vi "multi-function-fpga-main-Rev5.vi"(9 "stop":bool, 10 "Update":bool, 11 "fpga controls":T1[](array[typedef])=[{"Operation"=0, "Num. Steps"=0, "Begin"=0.0, "Step Size"=0.0, "Input - A"=0, "Input - B"=0, "Output - LO"=0.0, "Output - HI"=0.0, "Reset"=FALSE, "Analog Output"=0, "Trigger Input"=0, "Initialize To"=0, "Digital Inputs"=[0, 0, 0, 0, 0], "Output Values"=[0.0, 0.0, 0.0, 0.0, 0.0], "Num. Inputs"=4}, {"Operation"=0, "Num. Steps"=0, "Begin"=0.0, "Step Size"=0.0, "Input - A"=0, "Input - B"=0, "Output - LO"=0.0, "Output - HI"=0.0, "Reset"=FALSE, "Analog Output"=1, "Trigger Input"=0, "Initialize To"=0, "Digital Inputs"=[0, 0, 0, 0, 0], "Output Values"=[0.0, 0.0, 0.0, 0.0, 0.0], "Num. Inputs"=4}, {"Operation"=0, "Num. Steps"=0, "Begin"=0.0, "Step Size"=0.0, "Input - A"=0, "Input - B"=0, "Output - LO"=0.0, "Output - HI"=0.0, "Reset"=FALSE, "Analog Output"=2, "Trigger Input"=0, "Initialize To"=0, "Digital Inputs"=[0, 0, 0, 0, 0], "Output Values"=[0.0, 0.0, 0.0, 0.0, 0.0], "Num. Inputs"=4}, {"Operation"=0, "Num. Steps"=0, "Begin"=0.0, "Step Size"=0.0, "Input - A"=0, "Input - B"=0, "Output - LO"=0.0, "Output - HI"=0.0, "Reset"=FALSE, "Analog Output"=3, "Trigger Input"=0, "Initialize To"=0, "Digital Inputs"=[0, 0, 0, 0, 0], "Output Values"=[0.0, 0.0, 0.0, 0.0, 0.0], "Num. Inputs"=4}, {"Operation"=0, "Num. Steps"=0, "Begin"=0.0, "Step Size"=0.0, "Input - A"=0, "Input - B"=0, "Output - LO"=0.0, "Output - HI"=0.0, "Reset"=FALSE, "Analog Output"=4, "Trigger Input"=0, "Initialize To"=0, "Digital Inputs"=[0, 0, 0, 0, 0], "Output Values"=[0.0, 0.0, 0.0, 0.0, 0.0], "Num. Inputs"=4}, {"Operation"=0, "Num. Steps"=0, "Begin"=0.0, "Step Size"=0.0, "Input - A"=0, "Input - B"=0, "Output - LO"=0.0, "Output - HI"=0.0, "Reset"=FALSE, "Analog Output"=5, "Trigger Input"=0, "Initialize To"=0, "Digital Inputs"=[0, 0, 0, 0, 0], "Output Values"=[0.0, 0.0, 0.0, 0.0, 0.0], "Num. Inputs"=4}, {"Operation"=0, "Num. Steps"=0, "Begin"=0.0, "Step Size"=0.0, "Input - A"=0, "Input - B"=0, "Output - LO"=0.0, "Output - HI"=0.0, "Reset"=FALSE, "Analog Output"=6, "Trigger Input"=0, "Initialize To"=0, "Digital Inputs"=[0, 0, 0, 0, 0], "Output Values"=[0.0, 0.0, 0.0, 0.0, 0.0], "Num. Inputs"=4}, {"Operation"=0, "Num. Steps"=0, "Begin"=0.0, "Step Size"=0.0, "Input - A"=0, "Input - B"=0, "Output - LO"=0.0, "Output - HI"=0.0, "Reset"=FALSE, "Analog Output"=7, "Trigger Input"=0, "Initialize To"=0, "Digital Inputs"=[0, 0, 0, 0, 0], "Output Values"=[0.0, 0.0, 0.0, 0.0, 0.0], "Num. Inputs"=4}, {"Operation"=0, "Num. Steps"=0, "Begin"=0.0, "Step Size"=0.0, "Input - A"=0, "Input - B"=0, "Output - LO"=0.0, "Output - HI"=0.0, "Reset"=FALSE, "Analog Output"=8, "Trigger Input"=0, "Initialize To"=0, "Digital Inputs"=[0, 0, 0, 0, 0], "Output Values"=[0.0, 0.0, 0.0, 0.0, 0.0], "Num. Inputs"=4}, {"Operation"=0, "Num. Steps"=0, "Begin"=0.0, "Step Size"=0.0, "Input - A"=0, "Input - B"=0, "Output - LO"=0.0, "Output - HI"=0.0, "Reset"=FALSE, "Analog Output"=9, "Trigger Input"=0, "Initialize To"=0, "Digital Inputs"=[0, 0, 0, 0, 0], "Output Values"=[0.0, 0.0, 0.0, 0.0, 0.0], "Num. Inputs"=4}, {"Operation"=0, "Num. Steps"=0, "Begin"=0.0, "Step Size"=0.0, "Input - A"=0, "Input - B"=0, "Output - LO"=0.0, "Output - HI"=0.0, "Reset"=FALSE, "Analog Output"=10, "Trigger Input"=0, "Initialize To"=0, "Digital Inputs"=[0, 0, 0, 0, 0], "Output Values"=[0.0, 0.0, 0.0, 0.0, 0.0], "Num. Inputs"=4}, {"Operation"=0, "Num. Steps"=0, "Begin"=0.0, "Step Size"=0.0, "Input - A"=0, "Input - B"=0, "Output - LO"=0.0, "Output - HI"=0.0, "Reset"=FALSE, "Analog Output"=11, "Trigger Input"=0, "Initialize To"=0, "Digital Inputs"=[0, 0, 0, 0, 0], "Output Values"=[0.0, 0.0, 0.0, 0.0, 0.0], "Num. Inputs"=4}, {"Operation"=0, "Num. Steps"=0, "Begin"=0.0, "Step Size"=0.0, "Input - A"=0, "Input - B"=0, "Output - LO"=0.0, "Output - HI"=0.0, "Reset"=FALSE, "Analog Output"=12, "Trigger Input"=0, "Initialize To"=0, "Digital Inputs"=[0, 0, 0, 0, 0], "Output Values"=[0.0, 0.0, 0.0, 0.0, 0.0], "Num. Inputs"=4}, {"Operation"=0, "Num. Steps"=0, "Begin"=0.0, "Step Size"=0.0, "Input - A"=0, "Input - B"=0, "Output - LO"=0.0, "Output - HI"=0.0, "Reset"=FALSE, "Analog Output"=13, "Trigger Input"=0, "Initialize To"=0, "Digital Inputs"=[0, 0, 0, 0, 0], "Output Values"=[0.0, 0.0, 0.0, 0.0, 0.0], "Num. Inputs"=4}, {"Operation"=0, "Num. Steps"=0, "Begin"=0.0, "Step Size"=0.0, "Input - A"=0, "Input - B"=0, "Output - LO"=0.0, "Output - HI"=0.0, "Reset"=FALSE, "Analog Output"=14, "Trigger Input"=0, "Initialize To"=0, "Digital Inputs"=[0, 0, 0, 0, 0], "Output Values"=[0.0, 0.0, 0.0, 0.0, 0.0], "Num. Inputs"=4}, {"Operation"=0, "Num. Steps"=0, "Begin"=0.0, "Step Size"=0.0, "Input - A"=0, "Input - B"=0, "Output - LO"=0.0, "Output - HI"=0.0, "Reset"=FALSE, "Analog Output"=15, "Trigger Input"=0, "Initialize To"=0, "Digital Inputs"=[0, 0, 0, 0, 0], "Output Values"=[0.0, 0.0, 0.0, 0.0, 0.0], "Num. Inputs"=4}] {"Digital Inputs" items=["DIO0", "DIO1", "DIO2", "DIO3", "DIO4", "DIO5", "DIO6", "DIO7", "DIO8", "DIO9", "DIO10", "DIO11", "DIO12", "DIO13", "DIO14", "DIO15", "DIO16", "DIO17", "DIO18", "DIO19", "DIO20", "DIO21", "DIO22", "DIO23", "DIO24", "DIO25", "DIO26", "DIO27", "DIO28", "DIO29", "DIO30", "DIO31"]; "Initialize To" items=["Zero", "Begin Value"]; "Trigger Input" items=["DIO0", "DIO1", "DIO2", "DIO3", "DIO4", "DIO5", "DIO6", "DIO7", "DIO8", "DIO9", "DIO10", "DIO11", "DIO12", "DIO13", "DIO14", "DIO15", "DIO16", "DIO17", "DIO18", "DIO19", "DIO20", "DIO21", "DIO22", "DIO23", "DIO24", "DIO25", "DIO26", "DIO27", "DIO28", "DIO29", "DIO30", "DIO31"]; "Analog Output" items=["AO\\00", "AO\\01", "AO\\02", "AO\\03", "AO\\04", "AO\\05", "AO\\06", "AO\\07", "AO\\08", "AO\\09", "AO\\10", "AO\\11", "AO\\12", "AO\\13", "AO\\14", "AO\\15"]; "Input - B" items=["DIO0", "DIO1", "DIO2", "DIO3", "DIO4", "DIO5", "DIO6", "DIO7", "DIO8", "DIO9", "DIO10", "DIO11", "DIO12", "DIO13", "DIO14", "DIO15", "DIO16", "DIO17", "DIO18", "DIO19", "DIO20", "DIO21", "DIO22", "DIO23", "DIO24", "DIO25", "DIO26", "DIO27", "DIO28", "DIO29", "DIO30", "DIO31"]; "Input - A" items=["DIO0", "DIO1", "DIO2", "DIO3", "DIO4", "DIO5", "DIO6", "DIO7", "DIO8", "DIO9", "DIO10", "DIO11", "DIO12", "DIO13", "DIO14", "DIO15", "DIO16", "DIO17", "DIO18", "DIO19", "DIO20", "DIO21", "DIO22", "DIO23", "DIO24", "DIO25", "DIO26", "DIO27", "DIO28", "DIO29", "DIO30", "DIO31"]; "Operation" items=["OFF", "SWITCH", "AND GATE", "OR GATE", "ITERATION", "CUSTOM - 461nm Freq."]}) -> (2 "AO Values":fxp<+/-,20,5>[](array[numeric]), 3 "Loop Time (us)":u32)   [LabVIEW 2016]
uses:
  fpga_array_element.ctl
  <vilib>/rvi/Emulation/niFpgaGetClockAttributes.vi
  <vilib>/rvi/Emulation/niFpgaSctlEmulationGetInTimedLoop.vi
  <vilib>/rvi/Emulation/niFpgaEmulationReportErrorSimple.vi
  <vilib>/rvi/eio/common/nirviEmuTemplateMethod_errors.vi
  <vilib>/rvi/Emulation/niFpgaCriticalErrorInLSC.vi
  <vilib>/eio/EIONode/EIONode.xnode
panel:
  # "Boolean Operation Controls"
  # "Iteration Operation Controls"
  # "Custom Operation Controls"
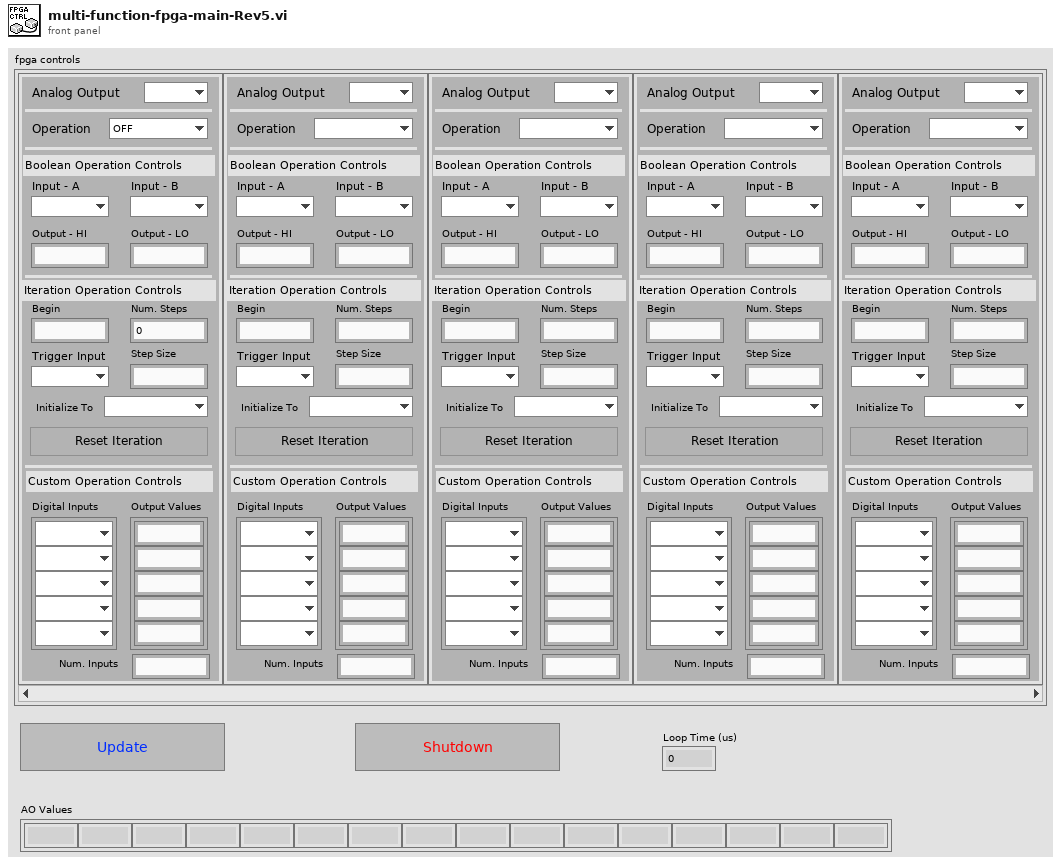
[diagram p1: front panel]
types:
  T1 = typedef "fpga_array_element.ctl" = cluster{"Operation":i16, "Num. Steps":u16, "Begin":fxp<+/-,20,5>, "Step Size":fxp<+/-,20,5>, "Input - A":i32, "Input - B":i32, "Output - LO":fxp<+/-,20,5>, "Output - HI":fxp<+/-,20,5>, "Reset":bool, "Analog Output":i32, "Trigger Input":i32, "Initialize To":i16, "Digital Inputs":i32[], "Output Values":fxp<+/-,20,5>[], "Num. Inputs":u16}
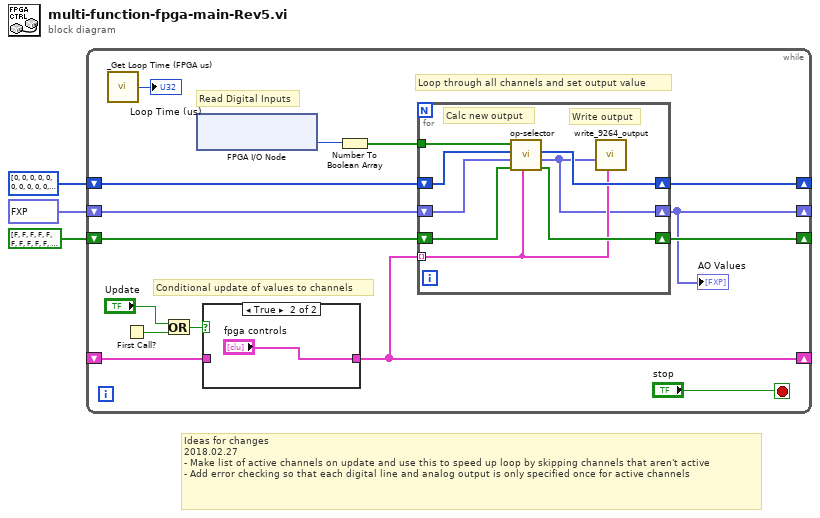
[diagram p0: block diagram]
diagram:
  # "Ideas for changes\n2018.02.27 \n- Make list of active channels on update and use this to speed up loop by skipping channels that aren't active \n- Add error checking so that each digital line and analog output is only specified once for active channels"
  n1 = while {
    shift-right: [w11] -> _
    shift-left: bool[] [FALSE, FALSE, FALSE, FALSE, FALSE, FALSE, FALSE, FALSE, FALSE, FALSE, FALSE, FALSE, FALSE, FALSE, FALSE, FALSE, FALSE, FALSE, FALSE, FALSE, FALSE, FALSE, FALSE, FALSE, FALSE, FALSE, FALSE, FALSE, FALSE, FALSE, FALSE, FALSE] -> [w13]
    shift-right: [w12] -> _
    shift-left: u16[] [0, 0, 0, 0, 0, 0, 0, 0, 0, 0, 0, 0, 0, 0, 0, 0] -> [w14]
    shift-right: [w15] -> _
    shift-left: _ -> [w17]
    shift-right: [w8] -> _
    shift-left: fxp<+/-,20,5>[] [0.0, 0.0, 0.0, 0.0, 0.0, 0.0, 0.0, 0.0, 0.0, 0.0, 0.0, 0.0, 0.0, 0.0, 0.0, 0.0] -> [w9]
    stop <- "stop" stop-if-true
    # "Loop through all channels and set output value"
    # "Read Digital Inputs"
    # "Conditional update of values to channels"
    n2 = call "_Get Loop Time (FPGA us).vi"() -> ("Loop Time (us)"=→"Loop Time (us)":u32)
    n3 = First Call?() -> (First Call?: T/F=w6:bool)
    n4 = Or(x="Update", y=w6) -> (x .or. y?=w7:bool)
    n5 = xnode "FPGA I/O Node"() -> ("Mod2/DIO31:0"=w16:u32)  [unwired: 1 in, 1 out]
    n6 = case shown="True" w7 {
      tunnel: [w27 "fpga controls"] -> w15
      tunnel: w17 -> [w27 _]
      frame False {
      }
      frame True {
      }
    }
    n7 = Number To Boolean Array(number=w16) -> (Boolean array=w4:bool[])
    n8 = for {
      tunnel: w15 -> [w20] mode=indexing
      tunnel: w4 -> [w26]
      shift-right: [w23] -> w12
      shift-left: w14 -> [w25]
      shift-right: [w19] -> w8
      shift-left: w9 -> [w21]
      shift-right: [w22] -> w11
      shift-left: w13 -> [w24]
      # "Write output"
      # "Calc new output"
      n9 = call "op-selector.vi"("Channel"=w20, "Prev DIO State"=w24, "Prev AO Values"=w21, "Iter Counter In"=w25, "Digital Input Value Array"=w26) -> ("Current DIO State"=w22:bool[], "New AO Values"=w19:fxp<+/-,20,5>[], "Iter Counter Out"=w23:u16[])  [unwired: 4 in]
      n10 = call "write_9264_output.vi"("Channel"=w20, "AO Values"=w19) -> ()  [unwired: 10 in]
    }
    "AO Values" <- w8
  }
